vi "S2C_FORNAX_Poly_TestBed.vi"() -> ()   [LabVIEW 2015]
uses:
  S2C_FORNAX_Poly_LaunchFornax.vi
  S2C_FORNAX_Poly_OpenSocket.vi
  S2C_FORNAX_Poly_BarcodeImageCommand.vi
  S2C_FORNAX_Poly_BoardIdCommand.vi
  S2C_FORNAX_Poly_DftAlarmCommand.vi
  S2C_FORNAX_Poly_DftAudioPlayCommand.vi
  S2C_FORNAX_Poly_DftInstrumentCommand.vi
  S2C_FORNAX_Poly_DftLogCommand.vi
  S2C_FORNAX_Poly_EmA2dCalDataCommand.vi
  S2C_FORNAX_Poly_EnergyParameterCommand.vi
  S2C_FORNAX_Poly_ExternalCommCommand.vi
  S2C_FORNAX_Poly_FeatureSettingsCommand.vi
  S2C_FORNAX_Poly_InstrumentSettingCommand.vi
  S2C_FORNAX_Poly_SystemConfigurationCommand.vi
  S2C_FORNAX_Poly_SystemSettingsCommand.vi
  S2C_FORNAX_Poly_TimeCommand.vi
  S2C_FORNAX_Poly_UserSettingsCommand.vi
  S2C_FORNAX_Poly_CloseFornax.vi
panel:
  out "Error Out":errorcluster
  in  "Error In":errorcluster
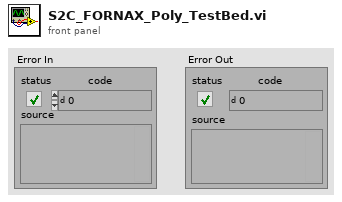
[diagram p1: front panel]
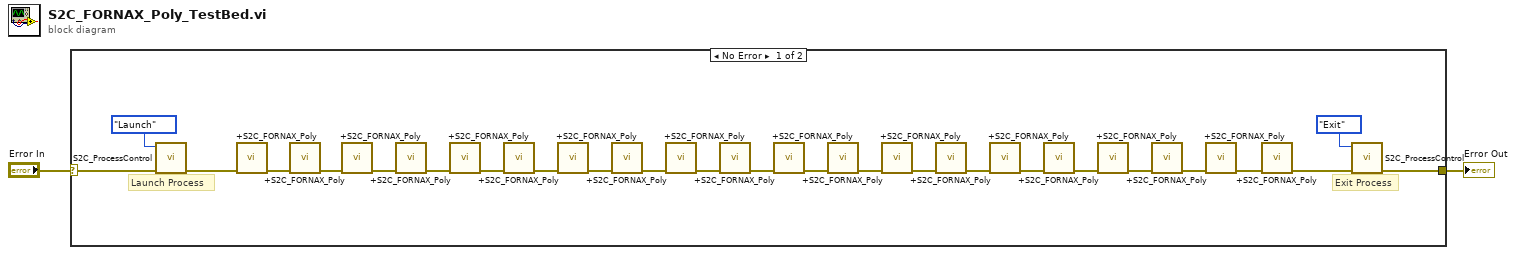
[diagram p0: block diagram]
diagram:
  n1 = case shown="No Error" "Error In" {
    selector: "Error In" -> [w8 w28]
    tunnel: [w25 w28] -> w1
    frame No Error {
      # "Exit Process"
      # "Launch Process"
      n2 = call "S2C_ProcessControl.vi"("Error In"=w8, "Action"=enum16{"Launch", "Exit"}."Launch") -> ("Error Out"=w7:errorcluster)  [unwired: 9 in]
      n3 = call-poly "+S2C_FORNAX_Poly.vi"("Error In"=w7) -> ("Error Out"=w6:errorcluster)  [unwired: 9 in, 1 out]
      n4 = call-poly "+S2C_FORNAX_Poly.vi"("Error In"=w6) -> ("Error Out"=w5:errorcluster)  [unwired: 9 in, 1 out]
      n5 = call-poly "+S2C_FORNAX_Poly.vi"("Error In"=w5) -> ("Error Out"=w24:errorcluster)  [unwired: 9 in, 1 out]
      n6 = call-poly "+S2C_FORNAX_Poly.vi"("Error In"=w24) -> ("Error Out"=w15:errorcluster)  [unwired: 9 in, 1 out]
      n7 = call-poly "+S2C_FORNAX_Poly.vi"("Error In"=w15) -> ("Error Out"=w14:errorcluster)  [unwired: 9 in, 1 out]
      n8 = call-poly "+S2C_FORNAX_Poly.vi"("Error In"=w14) -> ("Error Out"=w23:errorcluster)  [unwired: 9 in, 1 out]
      n9 = call-poly "+S2C_FORNAX_Poly.vi"("Error In"=w23) -> ("Error Out"=w13:errorcluster)  [unwired: 9 in, 1 out]
      n10 = call-poly "+S2C_FORNAX_Poly.vi"("Error In"=w13) -> ("Error Out"=w12:errorcluster)  [unwired: 9 in, 1 out]
      n11 = call-poly "+S2C_FORNAX_Poly.vi"("Error In"=w12) -> ("Error Out"=w22:errorcluster)  [unwired: 9 in, 1 out]
      n12 = call-poly "+S2C_FORNAX_Poly.vi"("Error In"=w22) -> ("Error Out"=w21:errorcluster)  [unwired: 9 in, 1 out]
      n13 = call-poly "+S2C_FORNAX_Poly.vi"("Error In"=w21) -> ("Error Out"=w20:errorcluster)  [unwired: 9 in, 1 out]
      n14 = call-poly "+S2C_FORNAX_Poly.vi"("Error In"=w20) -> ("Error Out"=w19:errorcluster)  [unwired: 9 in, 1 out]
      n15 = call-poly "+S2C_FORNAX_Poly.vi"("Error In"=w19) -> ("Error Out"=w11:errorcluster)  [unwired: 9 in, 1 out]
      n16 = call-poly "+S2C_FORNAX_Poly.vi"("Error In"=w11) -> ("Error Out"=w10:errorcluster)  [unwired: 9 in, 1 out]
      n17 = call-poly "+S2C_FORNAX_Poly.vi"("Error In"=w10) -> ("Error Out"=w18:errorcluster)  [unwired: 9 in, 1 out]
      n18 = call-poly "+S2C_FORNAX_Poly.vi"("Error In"=w18) -> ("Error Out"=w9:errorcluster)  [unwired: 9 in, 1 out]
      n19 = call-poly "+S2C_FORNAX_Poly.vi"("Error In"=w9) -> ("Error Out"=w17:errorcluster)  [unwired: 9 in, 1 out]
      n20 = call-poly "+S2C_FORNAX_Poly.vi"("Error In"=w17) -> ("Error Out"=w16:errorcluster)  [unwired: 9 in, 1 out]
      n21 = call-poly "+S2C_FORNAX_Poly.vi"("Error In"=w16) -> ("Error Out"=w4:errorcluster)  [unwired: 9 in, 1 out]
      n22 = call-poly "+S2C_FORNAX_Poly.vi"("Error In"=w4) -> ("Error Out"=w3:errorcluster)  [unwired: 9 in, 1 out]
      n23 = call "S2C_ProcessControl.vi"("Error In"=w3, "Action"=enum16{"Launch", "Exit"}."Exit") -> ("Error Out"=w25:errorcluster)  [unwired: 9 in]
    }
    frame Error {
    }
  }
  "Error Out" <- w1
